vi "VisionNetwork.vi"   [LabVIEW 2020]
uses:
  <vilib>/Rock Robotics/Network Tables/NT Read Number.vi
  VisionGlobals.vi
  <vilib>/Rock Robotics/WPI/ThirdParty/PhotonVisionLib/PhotonVisionLib.lvlib
  <vilib>/Rock Robotics/Network Tables/NT Write Number.vi
types:
  T1 = typedef "PhotonVisionLib.lvlib/PhotonPipelineResultType.ctl" = cluster{"TargetCount":i32, "Latency_MilliSec":dbl, "Targets":T2[]}
  T2 = typedef "PhotonVisionLib.lvlib/PhotonTrackedTargetType.ctl" = cluster{"Yaw":dbl, "Pitch":dbl, "Area":dbl, "Skew":dbl, "TargetCorners":T3[], "BestCameraToTarget":T4, "FiiducialId":i32, "AltCameraToTarget":T4, "PoseAmbiguity":dbl}
  T3 = typedef "PhotonVisionLib.lvlib/TargetCornerType.ctl" = cluster{"X":dbl, "Y":dbl}
  T4 = typedef "Trajectory_Library.lvlib/TRANSFORM3D.ctl" = cluster{"TRANSLATION3D":T5, "ROTATION3D":T6, "XF":bool}
  T5 = typedef "Trajectory_Library.lvlib/TRANSLATION3D.ctl" = cluster{"X":dbl, "Y":dbl, "Z":dbl}
  T6 = typedef "Trajectory_Library.lvlib/ROTATION3D.ctl" = cluster{"Q_quaternion":T7}
  T7 = typedef "Trajectory_Library.lvlib/QUATERNION.ctl" = cluster{"R":dbl, "V":dbl[]}
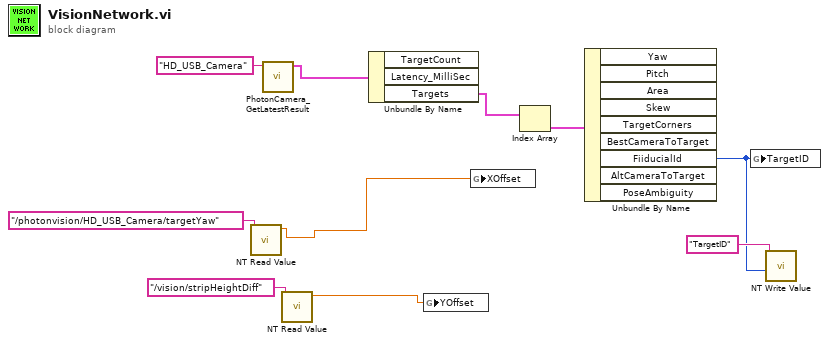
[diagram p0: block diagram]
diagram:
  n1 = call-poly <vilib>:"NT Read Value.vi"("Name"="/photonvision/HD_USB_Camera/targetYaw") -> ("Numeric"=w7:dbl)  [unwired: 9 in, 1 out]
  n2 = call <vilib>:"PhotonCamera_GetLatestResult.vi"("CameraName"="HD_USB_Camera") -> ("PipelineResult"=w5:T1)  [unwired: 9 in, 1 out]
  n3 = call-poly <vilib>:"NT Read Value.vi"("Name"="/vision/stripHeightDiff") -> ("Numeric"=w8:dbl)  [unwired: 9 in, 1 out]
  n4 = Unbundle By Name(w5) -> ("Targets"=w4:T2[])  [unwired: 2 out]
  n5 = global write "VisionGlobals.vi" "YOffset"(w8) -> ()
  n6 = global write "VisionGlobals.vi" "XOffset"(w7) -> ()
  n7 = Index Array(array=w4) -> (element=w3:T2)  [unwired: 1 in]
  n8 = Unbundle By Name(w3) -> ("FiiducialId"=w1:i32)  [unwired: 8 out]
  n9 = global write "VisionGlobals.vi" "TargetID"(w1) -> ()
  n10 = call-poly <vilib>:"NT Write Value.vi"("Numeric"=w1, "Name"="TargetID") -> ()  [unwired: 9 in, 1 out]
